vi "1_Image_To_ArrayU8.vi"(0 "Image Path":path, 7 "Buffer Src IN":T1, 11 "Error IN":errorcluster caption="Error in (no error)") -> (3 "Image Src OUT":T1(plugin-control), 4 "Array Src OUT":u8[](array[numeric]), 6 "Array Dst OUT":u8[](array[numeric]), 8 "Width or X":i32, 10 "Height or Y":i32, 15 "Error OUT":errorcluster)   [LabVIEW 2018]
doc: "It reads a source image (Type: BMP, TIFF, JPEG, JPEG2000, PNG or AIPD) and it returns the 1D Array U8 of the source image, the 1D array U8 that will save the destination image and the width and the height of the image. It receives the path of the source image and a buffer that reserves memory for the source image."
uses:
  <vilib>/vision/Image Controls.llb/IMAQ Image.ctl
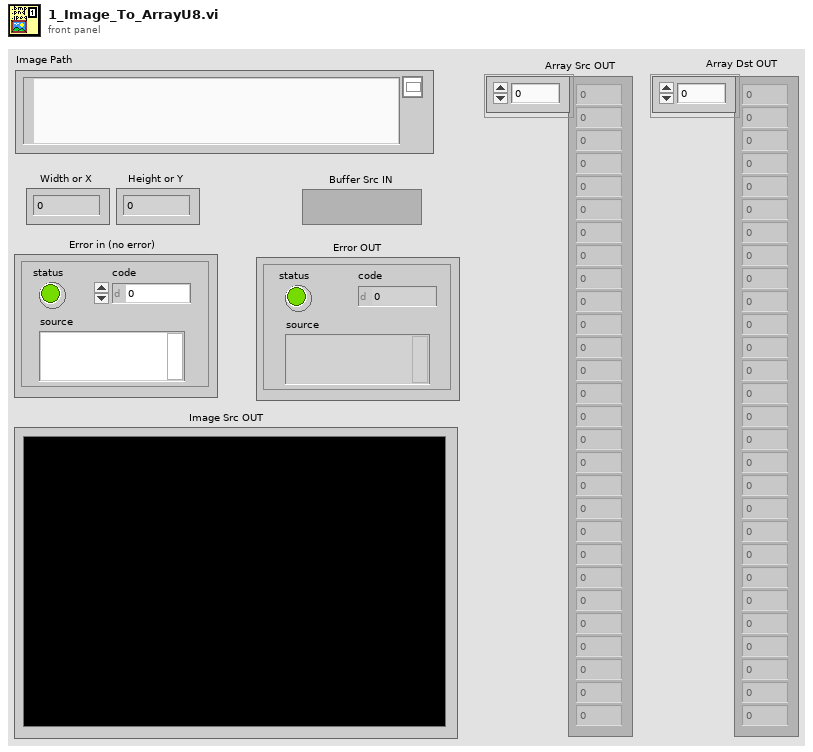
[diagram p1: front panel]
types:
  T1 = typedef "IMAQ Image.ctl" = refnum<image>
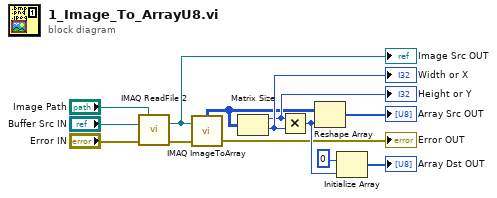
[diagram p0: block diagram]
diagram:
  n1 = call "IMAQ ReadFile 2"("File Path"="Image Path", "error in (no error)"="Error IN", "Image"="Buffer Src IN") -> ("error out"=w5:errorcluster, "Image Out"=w4:T1)  [unwired: 4 in, 3 out]
  "Image Src OUT" <- w4
  n2 = call "IMAQ ImageToArray"("error in (no error)"=w5, "Image"=w4) -> ("error out"=→"Error OUT":errorcluster, "Image Pixels (U8)"=w6:u8[][])  [unwired: 2 in, 3 out]
  n3 = Matrix Size(0:w6) -> (1:w7:i32, 2:w8:i32)
  "Height or Y" <- w7
  "Width or X" <- w8
  n4 = Multiply(x=w7, y=w8) -> (x*y=w10:i32)
  n5 = Reshape Array(w6, w10) -> (→"Array Src OUT":u8[])
  n6 = Initialize Array(u8 0 ("element"), w10) -> (→"Array Dst OUT":u8[])
